vi "Get Test Image.vi"(3 "queue in":refnum<queue>) -> (0 "no more images after this?":bool, 1 "Assembly Line Image":T1)   [LabVIEW 2023]
doc: "Get a board test image from the queue."
uses:
  Assembly Line Input.ctl
  Board Image.ctl
  Board Type Enum.ctl
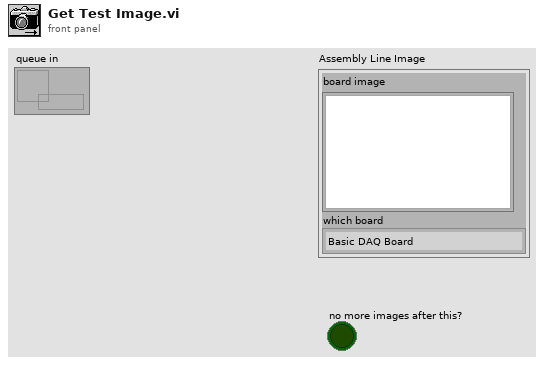
[diagram p1: front panel]
types:
  T1 = typedef "Assembly Line Input.ctl" = cluster{"board image":T2, "which board":T3}
  T2 = typedef "Board Image.ctl" = picture
  T3 = typedef "Board Type Enum.ctl" = enum16{"Basic DAQ Board", "Elite DAQ Board", "GPIB Board"}
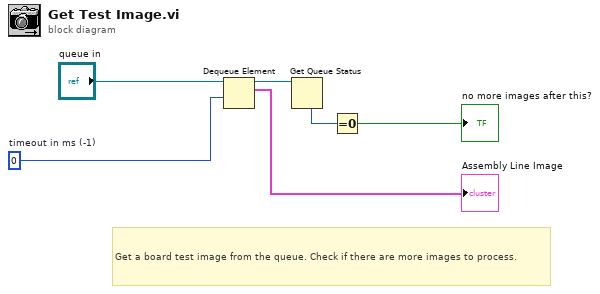
[diagram p0: block diagram]
diagram:
  w4 = 0  # timeout in ms (-1)
  # "Get a board test image from the queue. Check if there are more images to process."
  n1 = Dequeue Element(queue="queue in", timeout in ms (-1)=w4) -> (queue out=w3:refnum<queue>, element=→"Assembly Line Image":T1)  [unwired: 1 in, 2 out]
  n2 = Get Queue Status(queue=w3) -> (# elements in queue=w2:i32)  [unwired: 1 in, 8 out]
  n3 = Equal To 0?(x=w2) -> (x = 0?=→"no more images after this?":bool)
